vi "FT10_Connect Fornax.vi"(8 "error in (no error)":errorcluster, 10 "Fornax Executable Path":path=path "C:/Program Files (x86)/Medtronic/Fornax/x86/Fornax.exe", 11 "Message Handling Cluster in":T1) -> (0 "error out":errorcluster, 2 "Fornax Connected?":bool, 3 "Message Handling Cluster out":T1)   [LabVIEW 2024]
doc: "Sends command prompt scripts to connect to Fornax application. Fornax then talks to the generator."
uses:
  Controls/Control_Message Handling Cluster.ctl
  Controls/Control_M4X Connection.ctl
  Controls/Control_PXI-7854R FPGA Reference.ctl
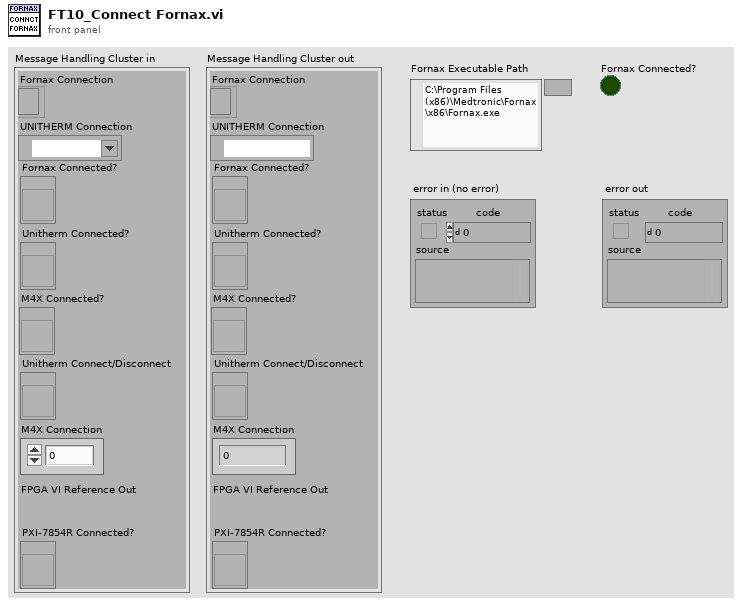
[diagram p1: front panel]
types:
  T1 = typedef "Control_Message Handling Cluster.ctl" = cluster{"Fornax Connection":refnum<k5>, "UNITHERM Connection":refnum<visa-resource-name>, "Fornax Connected?":refnum<vi>, "Unitherm Connected?":refnum<vi>, "M4X Connected?":refnum<vi>, "Unitherm Connect/Disconnect":refnum<vi>, "M4X Connection":T2, "PXI-7854R FPGA Reference":T3, "PXI-7854R Connected?":refnum<vi>}
  T2 = typedef "Control_M4X Connection.ctl" = u32
  T3 = typedef "Control_PXI-7854R FPGA Reference.ctl" = refnum<k20>
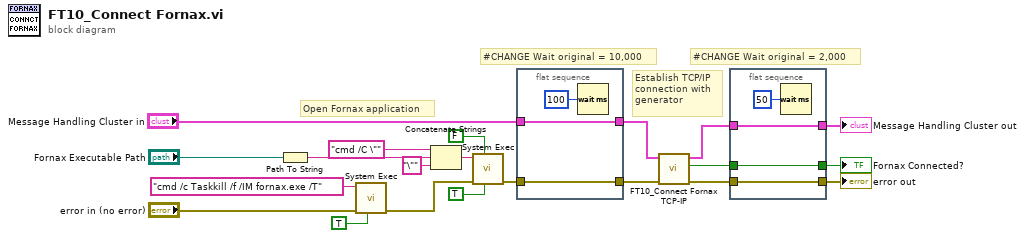
[diagram p0: block diagram]
diagram:
  # "Open Fornax application"
  # "Establish TCP/IP\nconnection with\ngenerator"
  # "#CHANGE Wait original = 2,000"
  # "#CHANGE Wait original = 10,000"
  n1 = Path To String(path="Fornax Executable Path") -> (string=w13:string)
  n2 = call <vilib>:"System Exec.vi"("run minimized? (F)"=TRUE, "error in (no error)"="error in (no error)", "command line"="cmd /c Taskkill /f /IM fornax.exe /T") -> ("error out"=w19:errorcluster)  [unwired: 5 in, 3 out]
  n3 = Concatenate Strings("cmd /C \"" ("string"), w13, "\"" ("string")) -> (w15:string)
  n4 = call <vilib>:"System Exec.vi"("run minimized? (F)"=TRUE, "wait until completion? (T)"=FALSE, "error in (no error)"=w19, "command line"=w15) -> ("error out"=w21:errorcluster)  [unwired: 4 in, 3 out]
  n5 = flat-sequence {
    tunnel: [w24] -> w8
    tunnel: w21 -> [w24]
    tunnel: [w22] -> w6
    tunnel: "Message Handling Cluster in" -> [w22]
    frame #0 {
      n6 = Wait (ms)(milliseconds to wait=u32 100) -> ()  [unwired: 1 out]
    }
  }
  n7 = call "FT10_Connect Fornax TCP-IP.vi"("error in (no error)"=w8, "Message Handling Cluster in"=w6) -> ("error out"=w7:errorcluster, "Fornax Connected?"=w2:bool, "Message Handling Cluster out"=w4:T1)  [unwired: 6 in, 1 out]
  n8 = flat-sequence {
    tunnel: [w28] -> w11
    tunnel: w7 -> [w28]
    tunnel: w4 -> [w26]
    tunnel: [w26] -> w3
    tunnel: w2 -> [w25]
    tunnel: [w25] -> w1
    frame #0 {
      n9 = Wait (ms)(milliseconds to wait=u32 50) -> ()  [unwired: 1 out]
    }
  }
  "error out" <- w11
  "Message Handling Cluster out" <- w3
  "Fornax Connected?" <- w1
